vi "ConfigLayouts.vi"(6 "Defer Updates? (True)":bool=TRUE, 7 "Tbl Refnum":refnum<vi>, 8 "error in (no error)":errorcluster, 9 "Col Array Refnum":refnum<vi>, 10 "Layout Ring Refnum":refnum<vi>) -> (0 "error out":errorcluster)   [LabVIEW 2013]
doc: "Manage existing and add new layouts. If a column is de-selected, it's width for the layout will be set to 0. The layout \"All\" is now protected and cannot be modified! In addition, the present SetList table view is populated in case the user wants to save an on-the-fly layout (created with \"Hide this column\".\nTo change column name, coloring, displayed width use Manage Devices... >>Edit.\n\nClearly, this VI requires read/write access to column data."
uses:
  TypeDefs/ColumnLayout_UI.ctl
  ColumnVIs/Column/Column.lvclass
  <vilib>/Utility/miscctls.llb/LVRowAndColumnTypeDef.ctl
panel:
  out "Non-user layouts":cluster{"String":string, "Value":i32}[](array[cluster])
  out "Trans LayoutInfo array":T1[][](array[typedef])
  in  "All On/Off Button":bool
  in  "RenameButton":bool
  in  "DeleteButton":bool caption="press cancel to undo!"
  in  "CancelButton":bool caption="Discard unsaved changes."
  in  "Save&CloseButton":bool
  in  "SaveButton":bool caption="need this button?"
  in  "NewButton":bool
  in  "Local Layout ring":i32(ring) caption="Select Layout:" items=["all off"]
  in  "ColLayout UI":T1[](array[typedef])
  # "Use the LED controls below to configure which columns appear in the selected layout. \n(Edit device to change label, color, width); Here: ON/OFF."
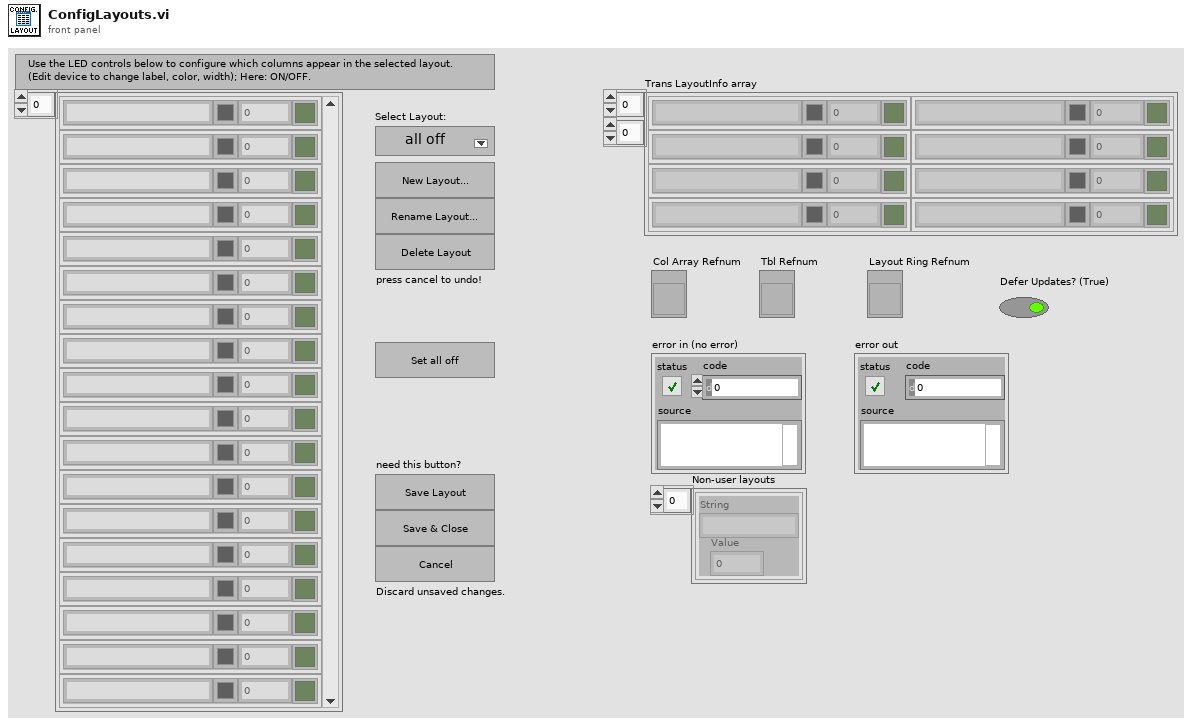
[diagram p1: front panel]
types:
  T1 = typedef "ColumnLayout_UI.ctl" = cluster{"Label":string, "Bgkd color":u32, "Width":u32, "Displayed?":bool}
  T2 = typedef "LVRowAndColumnTypeDef.ctl" = cluster{"Row":i32, "Column":i32}
  T3 = typedef "LVStringsAndValuesArrayTypeDef_I32.ctl" = cluster{"String":string, "Value":i32}[]
  T4 = enum8{"Enabled", "Disabled", "Disabled and Grayed Out"}
  T5 = typedef "ColumnLayoutCluster.ctl" = cluster{"Label":string, "Color":u32, "Width":u32, "[disp?]":bool[]}
  T6 = cluster{"Label":bool, "Bgkd color":bool, "Width":bool, "Displayed?":bool}[]
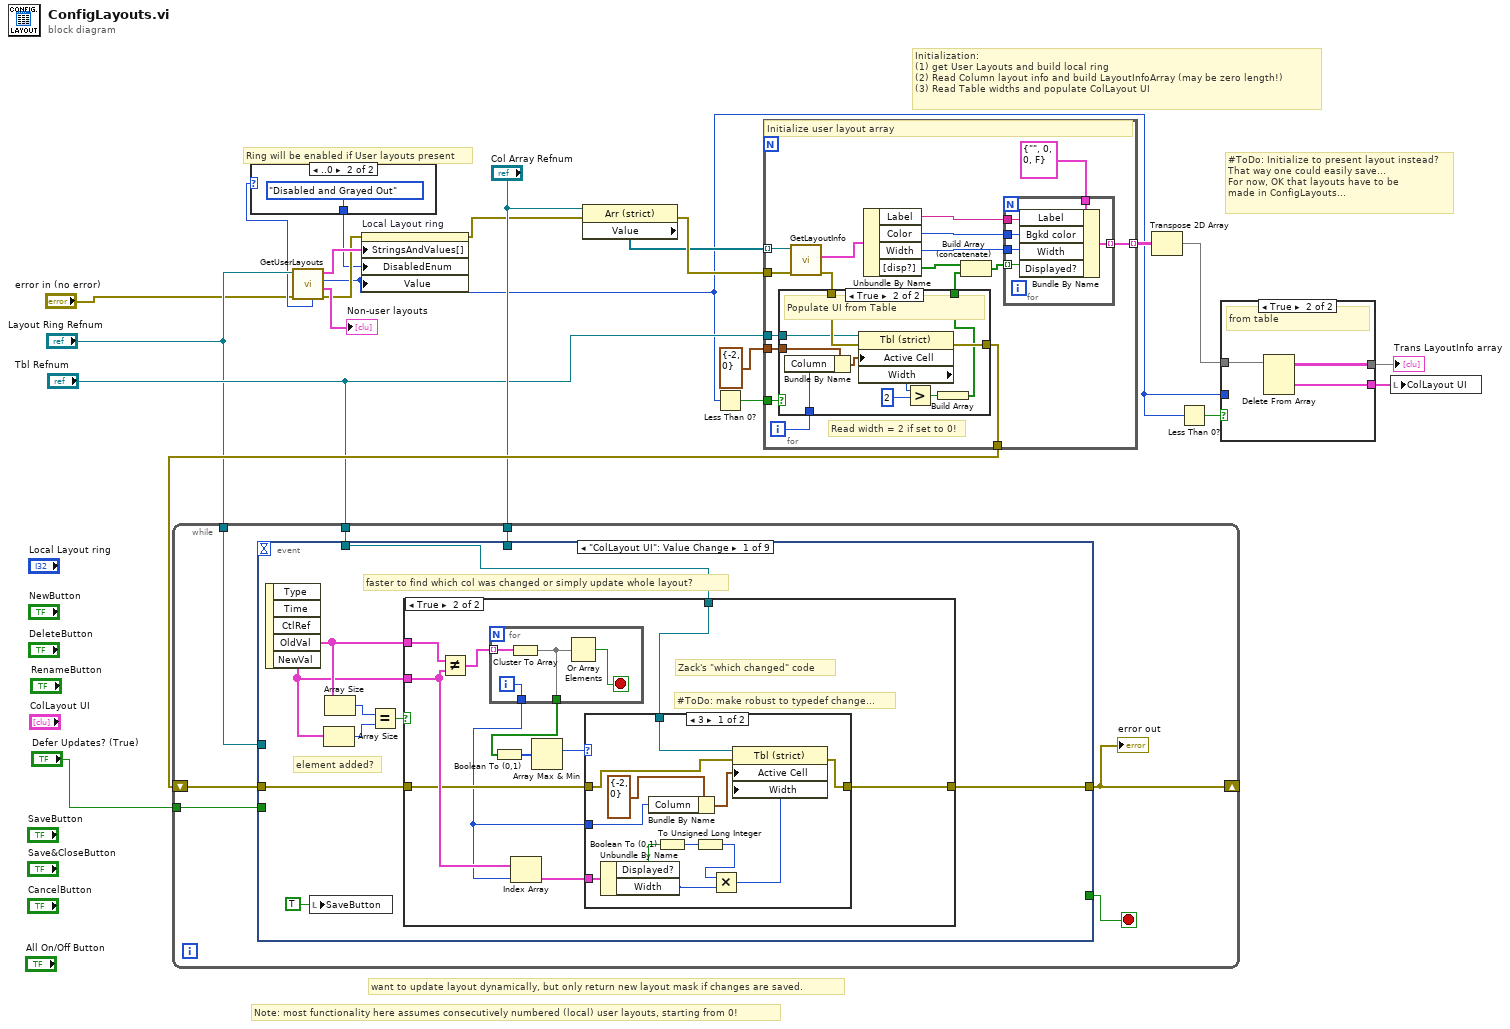
[diagram p0: block diagram]
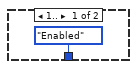
[diagram p2: hidden frame]
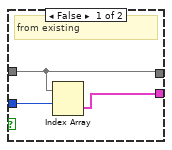
[diagram p3: hidden frame]
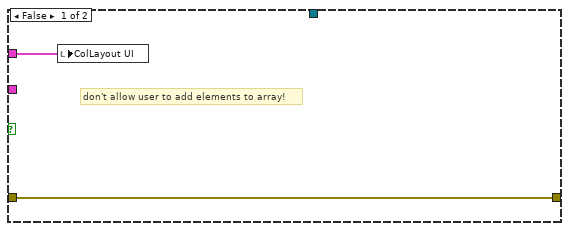
[diagram p4: hidden frame]
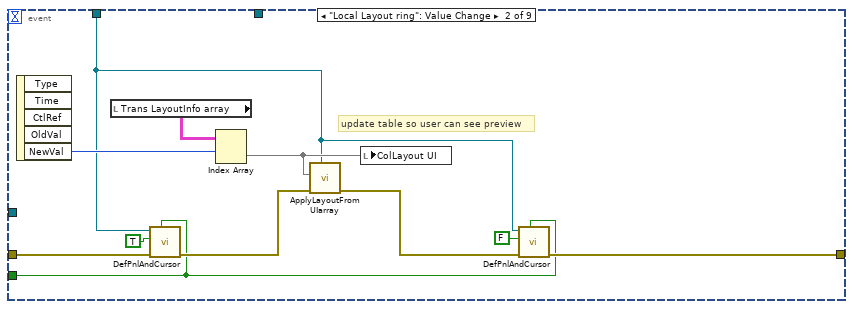
[diagram p6: hidden frame]
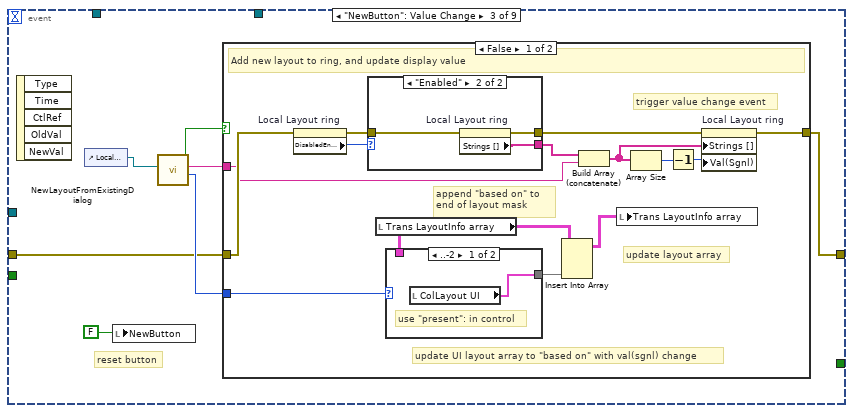
[diagram p7: hidden frame]
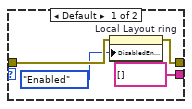
[diagram p8: hidden frame]
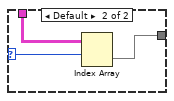
[diagram p9: hidden frame]
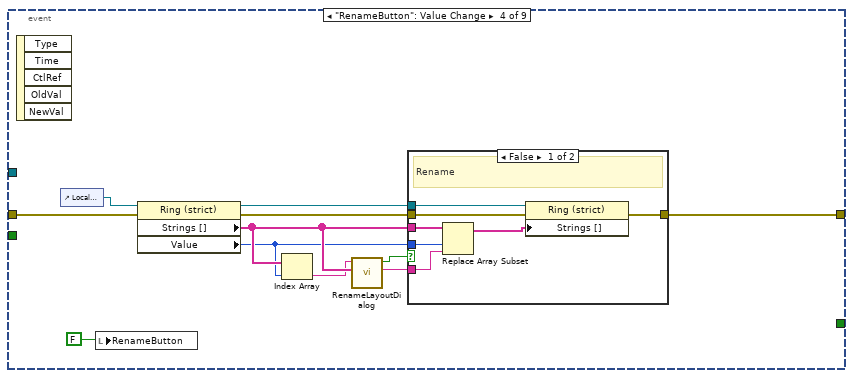
[diagram p11: hidden frame]
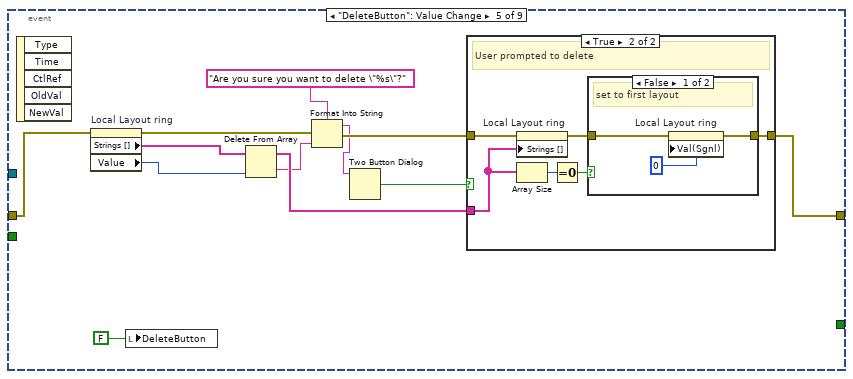
[diagram p13: hidden frame]
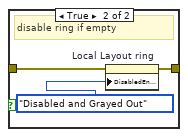
[diagram p15: hidden frame]
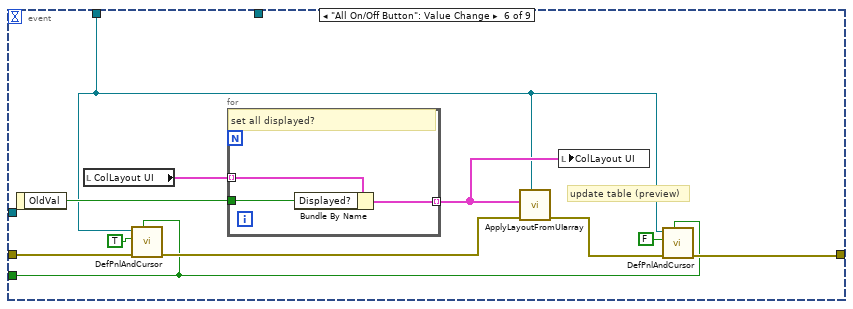
[diagram p16: hidden frame]
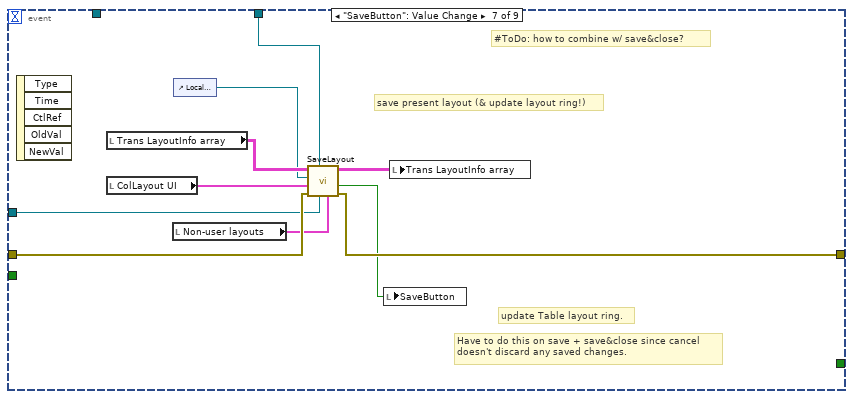
[diagram p17: hidden frame]
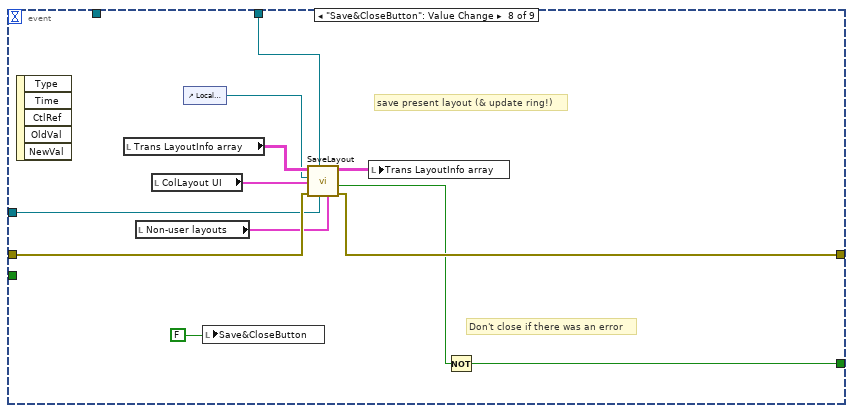
[diagram p18: hidden frame]
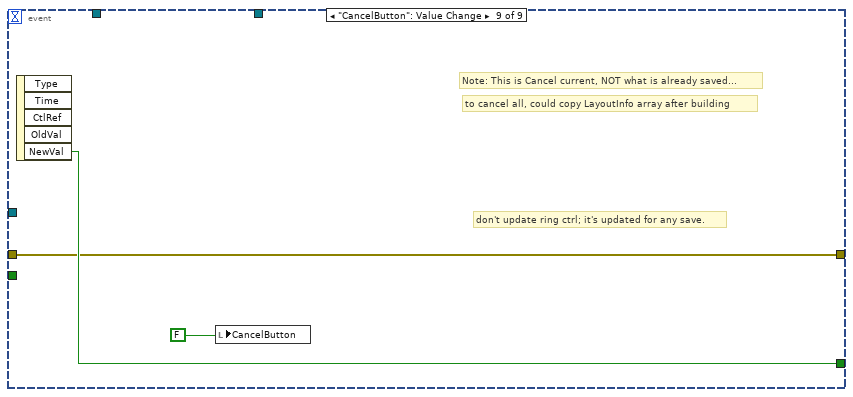
[diagram p19: hidden frame]
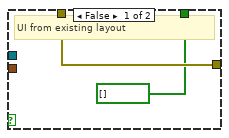
[diagram p20: hidden frame]
diagram:
  # "Ring will be enabled if User layouts present"
  # "Initialization:\n(1) get User Layouts and build local ring\n(2) Read Column layout info and build LayoutInfoArray (may be zero length!)\n(3) Read Table widths and populate ColLayout UI"
  # "Note: most functionality here assumes consecutively numbered (local) user layouts, starting from 0!"
  # "#ToDo: Initialize to present layout instead?\nThat way one could easily save...\nFor now, OK that layouts have to be \nmade in ConfigLayouts..."
  # "want to update layout dynamically, but only return new layout mask if changes are saved."
  n1 = call "GetUserLayouts.vi"("error in (no error)"="error in (no error)", "Layout Ring Refnum"="Layout Ring Refnum") -> ("error out"=w6:errorcluster, "Non-user Strings And Values []"=→"Non-user layouts":T3, "Value"=w2:i32, "User StringsAndValues[]"=w8:T3, "Num User Layouts"=w3:i32)  [unwired: 5 in]
  n2 = case shown="..0" w3 {
    tunnel: [T4."Enabled" ("Disabled") T4."Disabled and Grayed Out" ("Disabled")] -> w5
    frame 1.. {
    }
    frame ..0 {
    }
  }
  n3 = property on="Local Layout ring" class="Ring (strict)"(error in=w6, "StringsAndValues[]"=w8, "DisabledEnum"=w5, "Value"=w2) -> (error out=w4:errorcluster)  [unwired: 1 in, 1 out]
  n4 = property class="Arr (strict)"(reference="Col Array Refnum", error in=w4) -> (error out=w22:errorcluster, "Value"=w21:refnum<class "Column.lvclass">[])  [unwired: 1 out]
  n5 = Less Than 0?(x=w2) -> (x < 0?=w10:bool)
  n6 = for {
    tunnel: w21 -> [w40] mode=indexing
    tunnel: w22 -> [w41]
    tunnel: [w32] -> w20
    tunnel: [w34] -> w17 mode=indexing
    tunnel: T2 {"Row"=-2, "Column"=0} ("Active Cell:Active Cell") -> [w31]
    tunnel: "Tbl Refnum" -> [w29]
    tunnel: w10 -> [w25]
    i -> [w30]
    # "Read width = 2 if set to 0!"
    # "Initialize user layout array"
    n7 = call "GetLayoutInfo.vi"("error in (no error)"=w41, "Column in"=w40) -> ("error out"=w33:errorcluster, "Layout cluster"=w39:T5)  [unwired: 7 in, 1 out]
    n8 = case shown="True" w25 {
      tunnel: w33 -> [w43 w53]
      tunnel: [w43 w52] -> w32
      tunnel: w31 -> [_ w51]
      tunnel: w30 -> [_ w50]
      tunnel: w29 -> [_ w48]
      tunnel: [bool[] [] w46] -> w26
      frame False {
        # "UI from existing layout"
      }
      frame True {
        # "Populate UI from Table"
        n9 = Bundle By Name(cluster=w51, "Column"=w50) -> (w49:T2)
        n10 = property class="Tbl (strict)"(reference=w48, error in=w53, "Active Cell"=w49) -> (error out=w52:errorcluster, "Width"=w45:u32)  [unwired: 1 out]
        n11 = Greater?(x=w45, y=u32 2) -> (0:w47:bool)
        n12 = Build Array(w47) -> (w46:bool[])
      }
    }
    n13 = Unbundle By Name(w39) -> ("Label"=w37:string, "Color"=w36:u32, "Width"=w35:u32, "[disp?]"=w28:bool[])
    n14 = Build Array (concatenate)(w28, w26) -> (w27:bool[])
    n15 = for {
      tunnel: T1 {"Label"="", "Bgkd color"=0, "Width"=0, "Displayed?"=FALSE} ("Column Layout") -> [w59]
      tunnel: w37 -> [w58]
      tunnel: w36 -> [w57]
      tunnel: w35 -> [w56]
      tunnel: w27 -> [w55] mode=indexing
      tunnel: [w54] -> w34 mode=indexing
      n16 = Bundle By Name(cluster=w59, "Label"=w58, "Bgkd color"=w57, "Width"=w56, "Displayed?"=w55) -> (w54:T1)
    }
  }
  n17 = while {
    shift-right: [w64] -> _
    shift-left: w20 -> [w65]
    tunnel: "Tbl Refnum" -> [w63]
    tunnel: "Defer Updates? (True)" -> [w62]
    tunnel: "Col Array Refnum" -> [w61]
    tunnel: "Layout Ring Refnum" -> [w60]
    stop <- w66 stop-if-true
    n18 = event shown="[0] \"ColLayout UI\": Value Change" {
      selector: _ -> [_ _ _ _ _ _ _ _ _]
      dyn-events: _ -> [_ _ _ _ _ _ _ _ _]
      timeout: _ -> [_ _ _ _ _ _ _ _ _]
      tunnel: [_ _ _ _ _ _ _ w218 w232] -> w66
      tunnel: w65 -> [w70 w113 w118 w160 w175 w201 w217 w228 w230]
      tunnel: [w69 w109 w119 w157 w174 w198 w212 w223 w230] -> w64
      tunnel: w63 -> [w67 w108 _ _ _ w197 _ _ _]
      tunnel: w62 -> [_ w107 _ _ _ w194 _ _ _]
      tunnel: w61 -> [_ _ _ _ _ _ w215 w224 _]
      tunnel: w60 -> [_ _ _ _ _ _ w211 w221 _]
      event "ColLayout UI": Value Change {
        # "element added?"
        # "faster to find which col was changed or simply update whole layout?"
        n19 = event-data() -> ("OldVal"=w75:T1[], "NewVal"=w74:T1[])  [unwired: 1 in, 3 out]
        n20 = local write "SaveButton"(TRUE ("SaveButton")) -> ()
        n21 = Array Size(array=w74) -> (size(s)=w72:i32)
        n22 = Array Size(array=w75) -> (size(s)=w73:i32)
        n23 = Equal?(x=w73, y=w72) -> (x = y?=w71:bool)
        n24 = case shown="True" w71 {
          tunnel: w75 -> [w77 w87]
          tunnel: w74 -> [_ w86]
          tunnel: w70 -> [w76 w81]
          tunnel: [w76 w80] -> w69
          tunnel: w67 -> [_ w78]
          frame False {
            # "don't allow user to add elements to array!"
            n25 = local write "ColLayout UI"(w77) -> ()
          }
          frame True {
            # "#ToDo: make robust to typedef change..."
            # "Zack's \"which changed\" code"
            n26 = Not Equal?(x=w87, y=w86) -> (x != y?=w88:T6)
            n27 = for {
              tunnel: w88 -> [w102] mode=indexing
              tunnel: [w104] -> w84
              tunnel: [w103] -> w79
              i -> [w103]
              stop <- w105 stop-if-true
              n28 = Cluster To Array(cluster=w102) -> (array=w104:bool[])
              n29 = Or Array Elements(Boolean array=w104) -> (logical OR=w105:bool)
            }
            n30 = Boolean To (0,1)(Boolean=w84) -> (0, 1=w85:i16[])
            n31 = Index Array(array=w86, index=w79) -> (element=w82:T1)
            n32 = Array Max & Min(array=w85) -> (max index (indices)=w83:i32)  [unwired: 3 out]
            n33 = case shown="3" w83 {
              tunnel: w82 -> [w100 _]
              tunnel: w81 -> [w95 w101]
              tunnel: [w94 w101] -> w80
              tunnel: w79 -> [w90 _]
              tunnel: w78 -> [w89 _]
              frame 3 {
                n34 = Unbundle By Name(w100) -> ("Displayed?"=w99:bool, "Width"=w98:u32)
                n35 = Bundle By Name(cluster=T2 {"Row"=-2, "Column"=0} ("Active Cell:Active Cell"), "Column"=w90) -> (w91:T2)
                n36 = Boolean To (0,1)(Boolean=w99) -> (0, 1=w97:i16)
                n37 = To Unsigned Long Integer(number=w97) -> (unsigned 32bit integer=w96:u32)
                n38 = Multiply(x=w96, y=w98) -> (x*y=w93:u32)
                n39 = property class="Tbl (strict)"(reference=w89, error in=w95, "Active Cell"=w91, "Width"=w93) -> (error out=w94:errorcluster)  [unwired: 1 out]
              }
              frame Default {
                # "none of the other values\nare currently editable!"
              }
            }
          }
        }
      }
      event "Local Layout ring": Value Change {
        # "update table so user can see preview"
        n40 = event-data() -> ("NewVal"=w114:i32)  [unwired: 1 in, 4 out]
        n41 = local read "Trans LayoutInfo array"() -> (w116:T1[][])
        n42 = call "DefPnlAndCursor.vi"("AllowDefPan? (T)"=w107, "error in (no error)"=w113, "DeferPanUpdts?"=TRUE, "Tbl Ctrl Refnum"=w108) -> ("error out"=w112:errorcluster)  [unwired: 7 in]
        n43 = Index Array(array=w116, index (row)=w114) -> (element=w115:T1[])  [unwired: 1 in]
        n44 = call "ApplyLayoutFromUIarray.vi"("Tbl Refnum"=w108, "error in (no error)"=w112, "ColLayout Array"=w115) -> ("error out"=w110:errorcluster)  [unwired: 8 in]
        n45 = local write "ColLayout UI"(w115) -> ()
        n46 = call "DefPnlAndCursor.vi"("AllowDefPan? (T)"=w107, "error in (no error)"=w110, "DeferPanUpdts?"=FALSE, "Tbl Ctrl Refnum"=w108) -> ("error out"=w109:errorcluster)  [unwired: 7 in]
      }
      event "NewButton": Value Change {
        # "reset button"
        n47 = event-data() -> ()  [unwired: 1 in, 5 out]
        n48 = control-ref of="Local Layout ring"() -> (w123:refnum<vi>)
        n49 = local write "NewButton"(FALSE) -> ()
        n50 = call "NewLayoutFromExistingDialog.vi"("Layout Ring Refnum"=w123) -> ("Based on"=w120:i32, "New Layout name"=w121:string, "Cancelled?"=w122:bool)  [unwired: 8 in]
        n51 = case shown="False" w122 {
          tunnel: w121 -> [w127 _]
          tunnel: w120 -> [w130 _]
          tunnel: [w134 w149] -> w119
          tunnel: w118 -> [w129 w149]
          frame False {
            # "append \"based on\" to \nend of layout mask"
            # "trigger value change event"
            # "update UI layout array to \"based on\" with val(sgnl) change"
            # "update layout array"
            # "Add new layout to ring, and update display value"
            n52 = property on="Local Layout ring" class="Ring (strict)"(error in=w129) -> (error out=w128:errorcluster, "DisabledEnum"=w124:T4)  [unwired: 1 in, 1 out]
            n53 = case shown="\"Enabled\"" w124 {
              tunnel: [w139 w144] -> w137
              tunnel: w128 -> [w140 w143]
              tunnel: [string[] [] ("Strings []") w142] -> w126
              frame Default {
                n54 = property on="Local Layout ring" class="Ring (strict)"(error in=w140, "DisabledEnum"=T4."Enabled" ("Disabled")) -> (error out=w139:errorcluster)  [unwired: 1 in, 1 out]
              }
              frame "Enabled" {
                n55 = property on="Local Layout ring" class="Ring (strict)"(error in=w143) -> (error out=w144:errorcluster, "Strings []"=w142:string[])  [unwired: 1 in, 1 out]
              }
            }
            n56 = local read "Trans LayoutInfo array"() -> (w133:T1[][])
            n57 = case shown="..-2" w130 {
              selector: w130 -> [_ w146]
              tunnel: w133 -> [_ w148]
              tunnel: [w145 w147] -> w131
              frame ..-2 {
                # "use \"present\": in control"
                n58 = local read "ColLayout UI"() -> (w145:T1[])
              }
              frame Default {
                n59 = Index Array "Index Array"(array=w148, index (row)=w146) -> (element=w147:T1[])  [unwired: 1 in]
              }
            }
            n60 = Insert Into Array "Insert Into Array"(array=w133, new element=w131) -> (w132:T1[][])  [unwired: 2 in]
            n61 = Build Array (concatenate)(w126, w127) -> (w125:string[])
            n62 = local write "Trans LayoutInfo array"(w132) -> ()
            n63 = Array Size(array=w125) -> (size(s)=w135:i32)
            n64 = Decrement(x=w135) -> (x-1=w136:i32)
            n65 = property on="Local Layout ring" class="Ring (strict)"(error in=w137, "Strings []"=w125, "Val(Sgnl)"=w136) -> (error out=w134:errorcluster)  [unwired: 1 in, 1 out]
          }
          frame True {
            # "User cancelled."
          }
        }
      }
      event "RenameButton": Value Change {
        n66 = event-data() -> ()  [unwired: 1 in, 5 out]
        n67 = control-ref of="Local Layout ring"() -> (w159:refnum<vi>)
        n68 = local write "RenameButton"(FALSE) -> ()
        n69 = property class="Ring (strict)"(reference=w159, error in=w160) -> (reference out=w156:refnum<vi>, error out=w158:errorcluster, "Strings []"=w152:string[], "Value"=w151:i32)
        n70 = Index Array(array=w152, index=w151) -> (element=w150:string)
        n71 = call "RenameLayoutDialog.vi"("Strings []"=w152, "Change Layout Name:"=w150) -> ("New Layout name"=w155:string, "Cancelled?"=w154:bool)  [unwired: 8 in]
        n72 = case shown="False" w154 {
          tunnel: w158 -> [w167 w168]
          tunnel: [w166 w168] -> w157
          tunnel: w156 -> [w165 _]
          tunnel: w151 -> [w164 _]
          tunnel: w152 -> [w162 _]
          tunnel: w155 -> [w161 _]
          frame False {
            # "Rename"
            n73 = Replace Array Subset(array=w162, new element=w161, index=w164) -> (w163:string[])
            n74 = property class="Ring (strict)"(reference=w165, error in=w167, "Strings []"=w163) -> (error out=w166:errorcluster)  [unwired: 1 out]
          }
          frame True {
            # "User Cancelled"
          }
        }
      }
      event "DeleteButton": Value Change {
        n75 = event-data() -> ()  [unwired: 1 in, 5 out]
        n76 = property on="Local Layout ring" class="Ring (strict)"(error in=w175) -> (error out=w180:errorcluster, "Strings []"=w177:string[], "Value"=w169:i32)  [unwired: 1 in, 1 out]
        n77 = local write "DeleteButton"(FALSE) -> ()
        n78 = Delete From Array "Delete From Array"(array=w177, index=w169) -> (deleted portion=w170:string, array with subset deleted=w176:string[])  [unwired: 1 in]
        n79 = Format Into String(format string="Are you sure you want to delete \"%s\"?" ("message"), error in=w180, w170) -> (resulting string=w171:string, error out=w178:errorcluster)  [unwired: 1 in]
        n80 = Two Button Dialog(message=w171) -> (T button?=w179:bool)  [unwired: 2 in]
        n81 = case shown="True" w179 {
          tunnel: w178 -> [w181 w187]
          tunnel: w176 -> [_ w184]
          tunnel: [w181 w185] -> w174
          frame False {
            # "User Cancelled"
          }
          frame True {
            # "User prompted to delete"
            n82 = property on="Local Layout ring" class="Ring (strict)"(error in=w187, "Strings []"=w184) -> (error out=w186:errorcluster)  [unwired: 1 in, 1 out]
            n83 = Array Size(array=w184) -> (size(s)=w182:i32)
            n84 = Equal To 0?(x=w182) -> (x = 0?=w183:bool)
            n85 = case shown="False" w183 {
              tunnel: w186 -> [w190 w193]
              tunnel: [w189 w191] -> w185
              frame False {
                # "set to first layout"
                n86 = property on="Local Layout ring" class="Ring (strict)"(error in=w190, "Val(Sgnl)"=0 ("Value (Signaling)")) -> (error out=w189:errorcluster)  [unwired: 1 in, 1 out]
              }
              frame True {
                # "disable ring if empty"
                n87 = property on="Local Layout ring" class="Ring (strict)"(error in=w193, "DisabledEnum"=T4."Disabled and Grayed Out" ("Disabled")) -> (error out=w191:errorcluster)  [unwired: 1 in, 1 out]
              }
            }
          }
        }
      }
      event "All On/Off Button": Value Change {
        # "update table (preview)"
        n88 = event-data() -> ("OldVal"=w204:bool)  [unwired: 1 in]
        n89 = local read "ColLayout UI"() -> (w202:T1[])
        n90 = call "DefPnlAndCursor.vi"("AllowDefPan? (T)"=w194, "error in (no error)"=w201, "DeferPanUpdts?"=TRUE, "Tbl Ctrl Refnum"=w197) -> ("error out"=w200:errorcluster)  [unwired: 7 in]
        n91 = for {
          tunnel: w202 -> [w207] mode=indexing
          tunnel: [w206] -> w203 mode=indexing
          tunnel: w204 -> [w205]
          # "set all displayed?"
          n92 = Bundle By Name(cluster=w207, "Displayed?"=w205) -> (w206:T1)
        }
        n93 = call "ApplyLayoutFromUIarray.vi"("Tbl Refnum"=w197, "error in (no error)"=w200, "ColLayout Array"=w203) -> ("error out"=w199:errorcluster)  [unwired: 8 in]
        n94 = local write "ColLayout UI"(w203) -> ()
        n95 = call "DefPnlAndCursor.vi"("AllowDefPan? (T)"=w194, "error in (no error)"=w199, "DeferPanUpdts?"=FALSE, "Tbl Ctrl Refnum"=w197) -> ("error out"=w198:errorcluster)  [unwired: 7 in]
      }
      event "SaveButton": Value Change {
        # "#ToDo: how to combine w/ save&close?"
        # "Have to do this on save + save&close since cancel\ndoesn't discard any saved changes."
        # "update Table layout ring."
        # "save present layout (& update layout ring!)"
        n96 = event-data() -> ()  [unwired: 1 in, 5 out]
        n97 = local read "Trans LayoutInfo array"() -> (w214:T1[][])
        n98 = local read "ColLayout UI"() -> (w216:T1[])
        n99 = local read "Non-user layouts"() -> (w209:cluster{"String":string, "Value":i32}[])
        n100 = control-ref of="Local Layout ring"() -> (w210:refnum<vi>)
        n101 = call "SaveLayout.vi"("Non-user layouts"=w209, "Layout Ring Refnum"=w211, "Col Array Refnum"=w215, "error in (no error)"=w217, "ColLayout Array (empty)"=w216, "Local Layout ring"=w210, "Trans LayoutInfo array in"=w214) -> ("error out"=w212:errorcluster, "SaveError?"=w208:bool, "Trans LayoutInfo array out"=w213:T1[][])  [unwired: 2 in]
        n102 = local write "SaveButton"(w208) -> ()
        n103 = local write "Trans LayoutInfo array"(w213) -> ()
      }
      event "Save&CloseButton": Value Change {
        # "Don't close if there was an error"
        # "save present layout (& update ring!)"
        n104 = event-data() -> ()  [unwired: 1 in, 5 out]
        n105 = local read "Trans LayoutInfo array"() -> (w226:T1[][])
        n106 = local read "Non-user layouts"() -> (w220:cluster{"String":string, "Value":i32}[])
        n107 = local read "ColLayout UI"() -> (w227:T1[])
        n108 = control-ref of="Local Layout ring"() -> (w222:refnum<vi>)
        n109 = local write "Save&CloseButton"(FALSE) -> ()
        n110 = call "SaveLayout.vi"("Non-user layouts"=w220, "Layout Ring Refnum"=w221, "Col Array Refnum"=w224, "error in (no error)"=w228, "ColLayout Array (empty)"=w227, "Local Layout ring"=w222, "Trans LayoutInfo array in"=w226) -> ("error out"=w223:errorcluster, "SaveError?"=w219:bool, "Trans LayoutInfo array out"=w225:T1[][])  [unwired: 2 in]
        n111 = local write "Trans LayoutInfo array"(w225) -> ()
        n112 = Not(x=w219) -> (.not. x?=w218:bool)
      }
      event "CancelButton": Value Change {
        # "to cancel all, could copy LayoutInfo array after building"
        # "Note: This is Cancel current, NOT what is already saved..."
        # "don't update ring ctrl; it's updated for any save."
        n113 = event-data() -> ("NewVal"=w232:bool)  [unwired: 1 in, 4 out]
        n114 = local write "CancelButton"(FALSE) -> ()
      }
    }
    "error out" <- w64
  }
  n115 = Transpose 2D Array(2D array=w17) -> (transposed array=w14:T1[][])
  n116 = Less Than 0?(x=w2) -> (x < 0?=w11:bool)
  n117 = case shown="True" w11 {
    tunnel: w14 -> [w235 w238]
    tunnel: [w235 w237] -> w13
    tunnel: [w234 w236] -> w12
    tunnel: w2 -> [w233 _]
    frame False {
      # "from existing"
      n118 = Index Array(array=w235, index (row)=w233) -> (element=w234:T1[])  [unwired: 1 in]
    }
    frame True {
      # "from table"
      n119 = Delete From Array(array=w238) -> (deleted portion=w236:T1[], array with subset deleted=w237:T1[][])  [unwired: 3 in]
    }
  }
  "Trans LayoutInfo array" <- w13
  n120 = local write "ColLayout UI"(w12) -> ()
